vi "Main v2.vi"(0 "PID On":bool) -> (5 "Total (V)":dbl[](array[slide]) scale=-8.0..8.0, 6 "Force (N)":T2(graph)={"M1 ref force"=19.690402476780186, "M2 ref force"=19.690402476780186, "M1 mes force"=5.466389475814116, "M2 mes force"=1.4423805363163493})   [LabVIEW 2021]
uses:
  <vilib>/addons/control/pid/NI_PID_pid.lvlib
  <vilib>/platform/TimedLoop/XDataNode/XDataNode.xnode
  <vilib>/Platform/TimedLoop/XDataNode/nitl_modes.ctl
  <vilib>/Platform/TimedLoop/XDataNode/XDNodeRunTimeDep.lvlib
  <vilib>/Platform/TimedLoop/XDataNode/wakeup.ctl
  <vilib>/Platform/TimedLoop/XDataNode/timing_clust.ctl
  <vilib>/Analysis/NI_AALBase.lvlib
  <vilib>/DAQmx/configure/timing.llb/DAQmx Timing (Sample Clock).vi
  <vilib>/DAQmx/create/channels.llb/DAQmx Create Channel (DO-Digital Output).vi
  <vilib>/DAQmx/create/channels.llb/DAQmx Create Channel (AO-Voltage-Basic).vi
  <vilib>/DAQmx/create/channels.llb/DAQmx Create Channel (AI-Voltage-Basic).vi
  <vilib>/Analysis/baseanly.llb/Real Dot Product.vi
  <vilib>/DAQmx/write.llb/DAQmx Write (Digital 1D Bool 1Chan 1Samp).vi
  <vilib>/DAQmx/write.llb/DAQmx Write (Analog 1D DBL NChan 1Samp).vi
  <vilib>/addons/control/pid/pid.llb/PID (DBL).vi
panel:
  out "Period":i64
  out "Finished Late? [i-1]":bool
  in  "operation (0:open)":T1(ring)
  in  "Tab Control 2":enum32{"Start", "Trajectory", "RBF"}(tab)
  in  "Encoder":bool
  in  "Loadcell":bool
  in  "Set Tension":dbl=7.0
  in  "Motor Enable":bool[](array[boolean])=[FALSE, FALSE]
  in  "x":cluster{"Number":i32, "x_0":dbl, "x_f":dbl}={"Number"=20, "x_0"=0.0, "x_f"=500.0}
  in  "RBF":cluster{"STD":dbl, "Number":i32}={"STD"=150.0, "Number"=3}
  out "Weights":dbl[](array[numeric])=[3.49, 8.71, 7.36]
  out "Output":dbl(slide)=5.690310910676771 scale=0.0..10.0
  in  "Traj Start":i32(knob) scale=0.0..2.0
  in  "Tab Control":enum32{"Page 1", "Page 2"}(tab)
  out "XY Graph":cluster{dbl[], dbl[]}[](graph)=[{[0.0, 26.31578947368421, 52.63157894736842, 78.94736842105263, 105.26315789473684, 131.57894736842104, 157.89473684210526, 184.21052631578945, 210.52631578947367, 236.8421052631579, 263.1578947368421, 289.4736842105263, 315.7894736842105, 342.10526315789474, 368.4210526315789, 394.7368421052631, 421.05263157894734, 447.36842105263156, 473.6842105263158, 499.99999999999994], [3.49, 3.4367023266816097, 3.2816434014183695, 3.038602121132399, 2.728282054650678, 2.375405053956736, 2.0054833734466047, 1.6418498415053318, 1.303409208366113, 1.0033700058366293, 0.7489872481878055, 0.5421515616003525, 0.3805397094919775, 0.25900743528896036, 0.1709454164658713, 0.10940462192952286, 0.06789641734177898, 0.040859309931447936, 0.023843399552483855, 0.013492061286760112]}, {[0.0, 26.31578947368421, 52.63157894736842, 78.94736842105263, 105.26315789473684, 131.57894736842104, 157.89473684210526, 184.21052631578945, 210.52631578947367, 236.8421052631579, 263.1578947368421, 289.4736842105263, 315.7894736842105, 342.10526315789474, 368.4210526315789, 394.7368421052631, 421.05263157894734, 447.36842105263156, 473.6842105263158, 499.99999999999994], [2.1718577384502504, 2.86506550054527, 3.664972461281408, 4.546109122932967, 5.4681696051074065, 6.377890766498874, 7.213485399786169, 7.9112701950597755, 8.413568935864594, 8.676554069284796, 8.676554069284796, 8.413568935864594, 7.911270195059776, 7.213485399786169, 6.377890766498877, 5.468169605107408, 4.546109122932969, 3.6649724612814083, 2.86506550054527, 2.1718577384502518]}, {[0.0, 26.31578947368421, 52.63157894736842, 78.94736842105263, 105.26315789473684, 131.57894736842104, 157.89473684210526, 184.21052631578945, 210.52631578947367, 236.8421052631579, 263.1578947368421, 289.4736842105263, 315.7894736842105, 342.10526315789474, 368.4210526315789, 394.7368421052631, 421.05263157894734, 447.36842105263156, 473.6842105263158, 499.99999999999994], [0.028453172226519864, 0.050282928569135, 0.08616748455457215, 0.14318556780386613, 0.23072149495738908, 0.3605038009136996, 0.5462162532168332, 0.8025135420805027, 1.1433339522574764, 1.5795261165221341, 2.1159894678961577, 2.748736897872375, 3.462468433661673, 4.22932883340029, 5.009450199748302, 5.753626338747561, 6.408054903018468, 6.920600411014096, 7.247601468302764, 7.36]}, {[0.0, 26.31578947368421, 52.63157894736842, 78.94736842105263, 105.26315789473684, 131.57894736842104, 157.89473684210526, 184.21052631578945, 210.52631578947367, 236.8421052631579, 263.1578947368421, 289.4736842105263, 315.7894736842105, 342.10526315789474, 368.4210526315789, 394.7368421052631, 421.05263157894734, 447.36842105263156, 473.6842105263158, 499.99999999999994], [5.690310910676771, 6.352050755796014, 7.03278334725435, 7.727896811869232, 8.427173154715474, 9.11379962136931, 9.765185026449608, 10.35563357864561, 10.860312096488185, 11.259450191643559, 11.54153078536876, 11.704457395337322, 11.754278338213426, 11.701821668475418, 11.55828638271305, 11.331200565784492, 11.022060443293217, 10.626432182226953, 10.136510368400518, 9.545349799737012]}]
  out "Position (mm)":cluster{"Position":dbl, "ref_x (mm)":dbl}(graph)={"Position"=75.7275182286212, "ref_x (mm)"=0.0}
  in  "RBF":bool
  out "Speed (RPM)":dbl[](array[knob]) scale=-200.0..200.0
  in  "Set Point":dbl(slide)=19.690402476780186 scale=0.0..40.0
  in  "stop":bool
  in  "Tab Control 3":enum32{"Page 1", "Page 3", "Page 4", "Page 2"}(tab)=enum."Page 2"
  in  "PID gains":T3 {"derivative time (Td, min)" format="%.3f"; "integral time (Ti, min)" format="%.3f"; "proportional gain (Kc)" format="%.3f"}
  in  "Pos Control":bool
  out "output":dbl(knob)=-0.0 scale=-40.0..40.0
  in  "Gains":T4(array[cluster])=[{"proportional gain (Kc)"=0.17, "integral time (Ti, min)"=0.0, "derivative time (Td, min)"=0.0}, {"proportional gain (Kc)"=0.17, "integral time (Ti, min)"=0.0, "derivative time (Td, min)"=0.0}] {"derivative time (Td, min)" format="%.3f"; "integral time (Ti, min)" format="%.3f"; "proportional gain (Kc)" format="%.3f"}
  out "PID (V)":dbl[](array[slide])=[2.4180822101642323, 1.0] scale=-8.0..8.0
  # "FORCE"
  # "TRAJECTORY"
  # "INITIALIZE"
  # "TUNE"
  # "MONITOR"
  # "DEVEL"
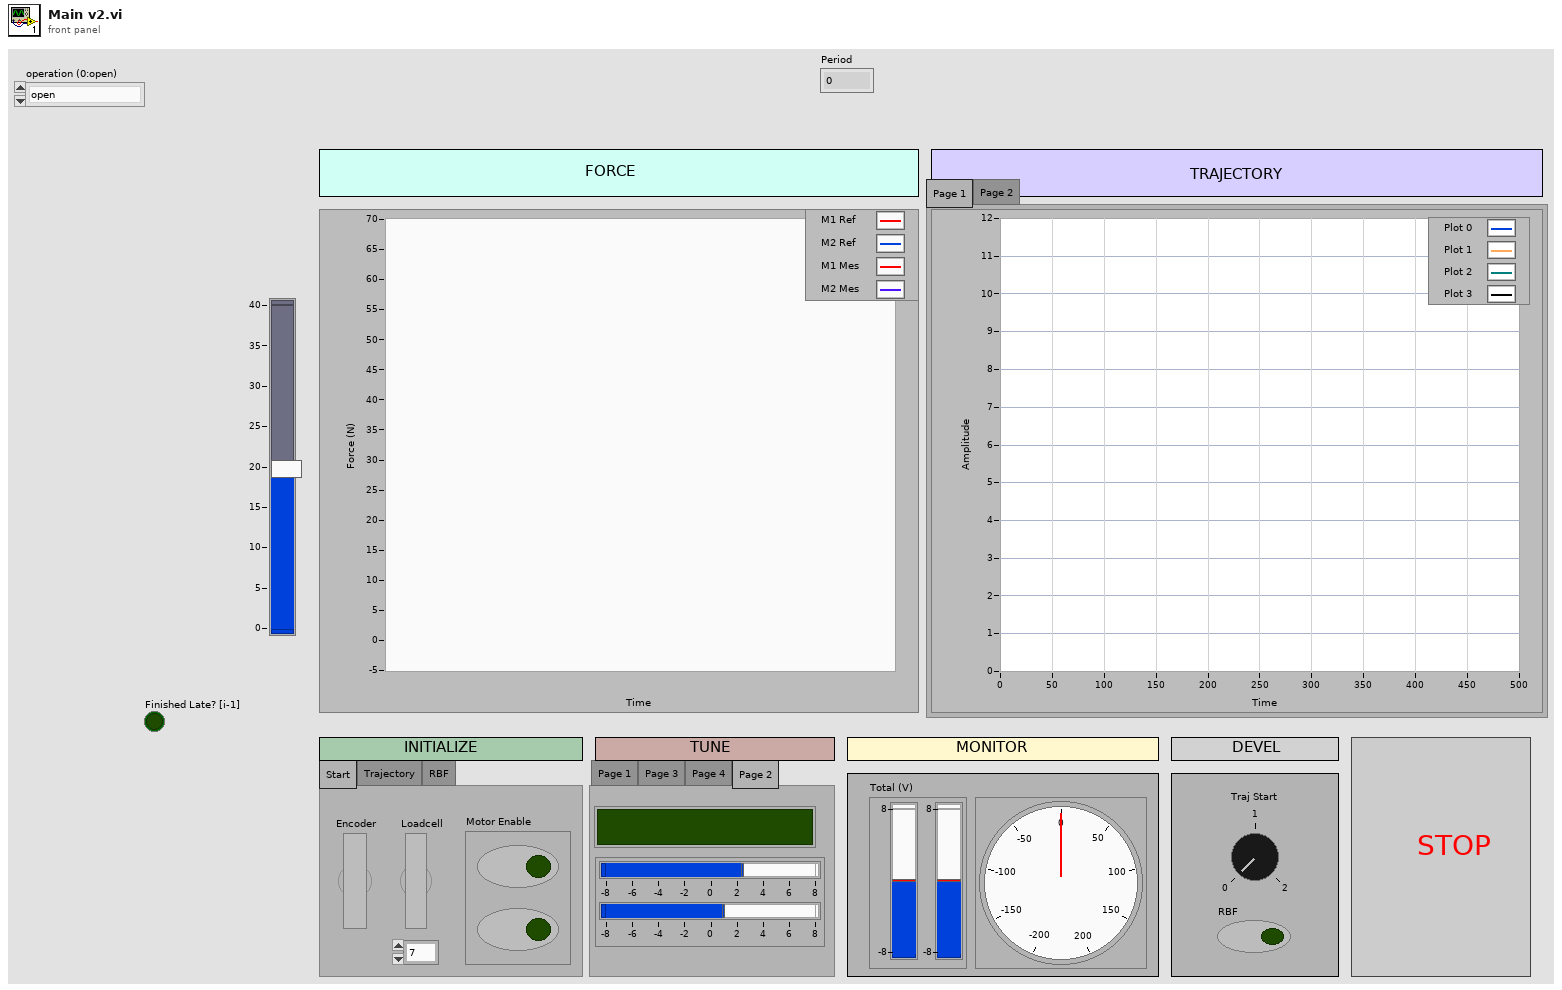
[diagram p1: front panel]
types:
  T1 = enum16{"open", "open or create", "create or replace", "create", "open (read-only)"}
  T2 = cluster{"M1 ref force":dbl, "M2 ref force":dbl, "M1 mes force":dbl, "M2 mes force":dbl}
  T3 = cluster{"proportional gain (Kc)":dbl, "integral time (Ti, min)":dbl, "derivative time (Td, min)":dbl}
  T4 = cluster{"proportional gain (Kc)":dbl, "integral time (Ti, min)":dbl, "derivative time (Td, min)":dbl}[]
  T5 = typedef "XDNodeRunTimeDep.lvlib/timing_clust.ctl" = cluster{"Expected End [f-1]":u64, "Actual End [f-1]":u64, "Finished Late? [f-1]":bool, "Expected End [i-1]":u64, "Actual End [i-1]":u64, "Finished Late? [i-1]":bool, "Expected Start [i]":u64, "Actual Start [i]":u64, "Expected Start [f]":u64, "Actual Start [f]":u64, "Source Name":string, "Structure Name":string, "Period":i64, "Deadline":i64, "Offset":i64, "Start":i64, "Priority":i32, "Timeout":i32, "Mode":T6, "Wakeup Reason":T7, "Error":errorcluster, "Source Type":string, "Secondary Source Type":string, "Global End Time":u64, "Global Start Time":u64, "Frame Duration":u64, "Iteration Duration":u64, "Assigned CPU":i32, "I/O Scan Engine Mode":u32}
  T6 = typedef "XDNodeRunTimeDep.lvlib/nitl_modes.ctl" = enum32{"No Change", "Process missed periods, maintain original phase", "Discard missed periods, maintain original phase", "Process missed periods, ignore original phase", "Discard missed periods, ignore original phase"}
  T7 = typedef "XDNodeRunTimeDep.lvlib/wakeup.ctl" = enum32{"Normal", "Aborted", "Asynchronous wakeup", "Timing source error", "Timed loop error", "Timeout"}
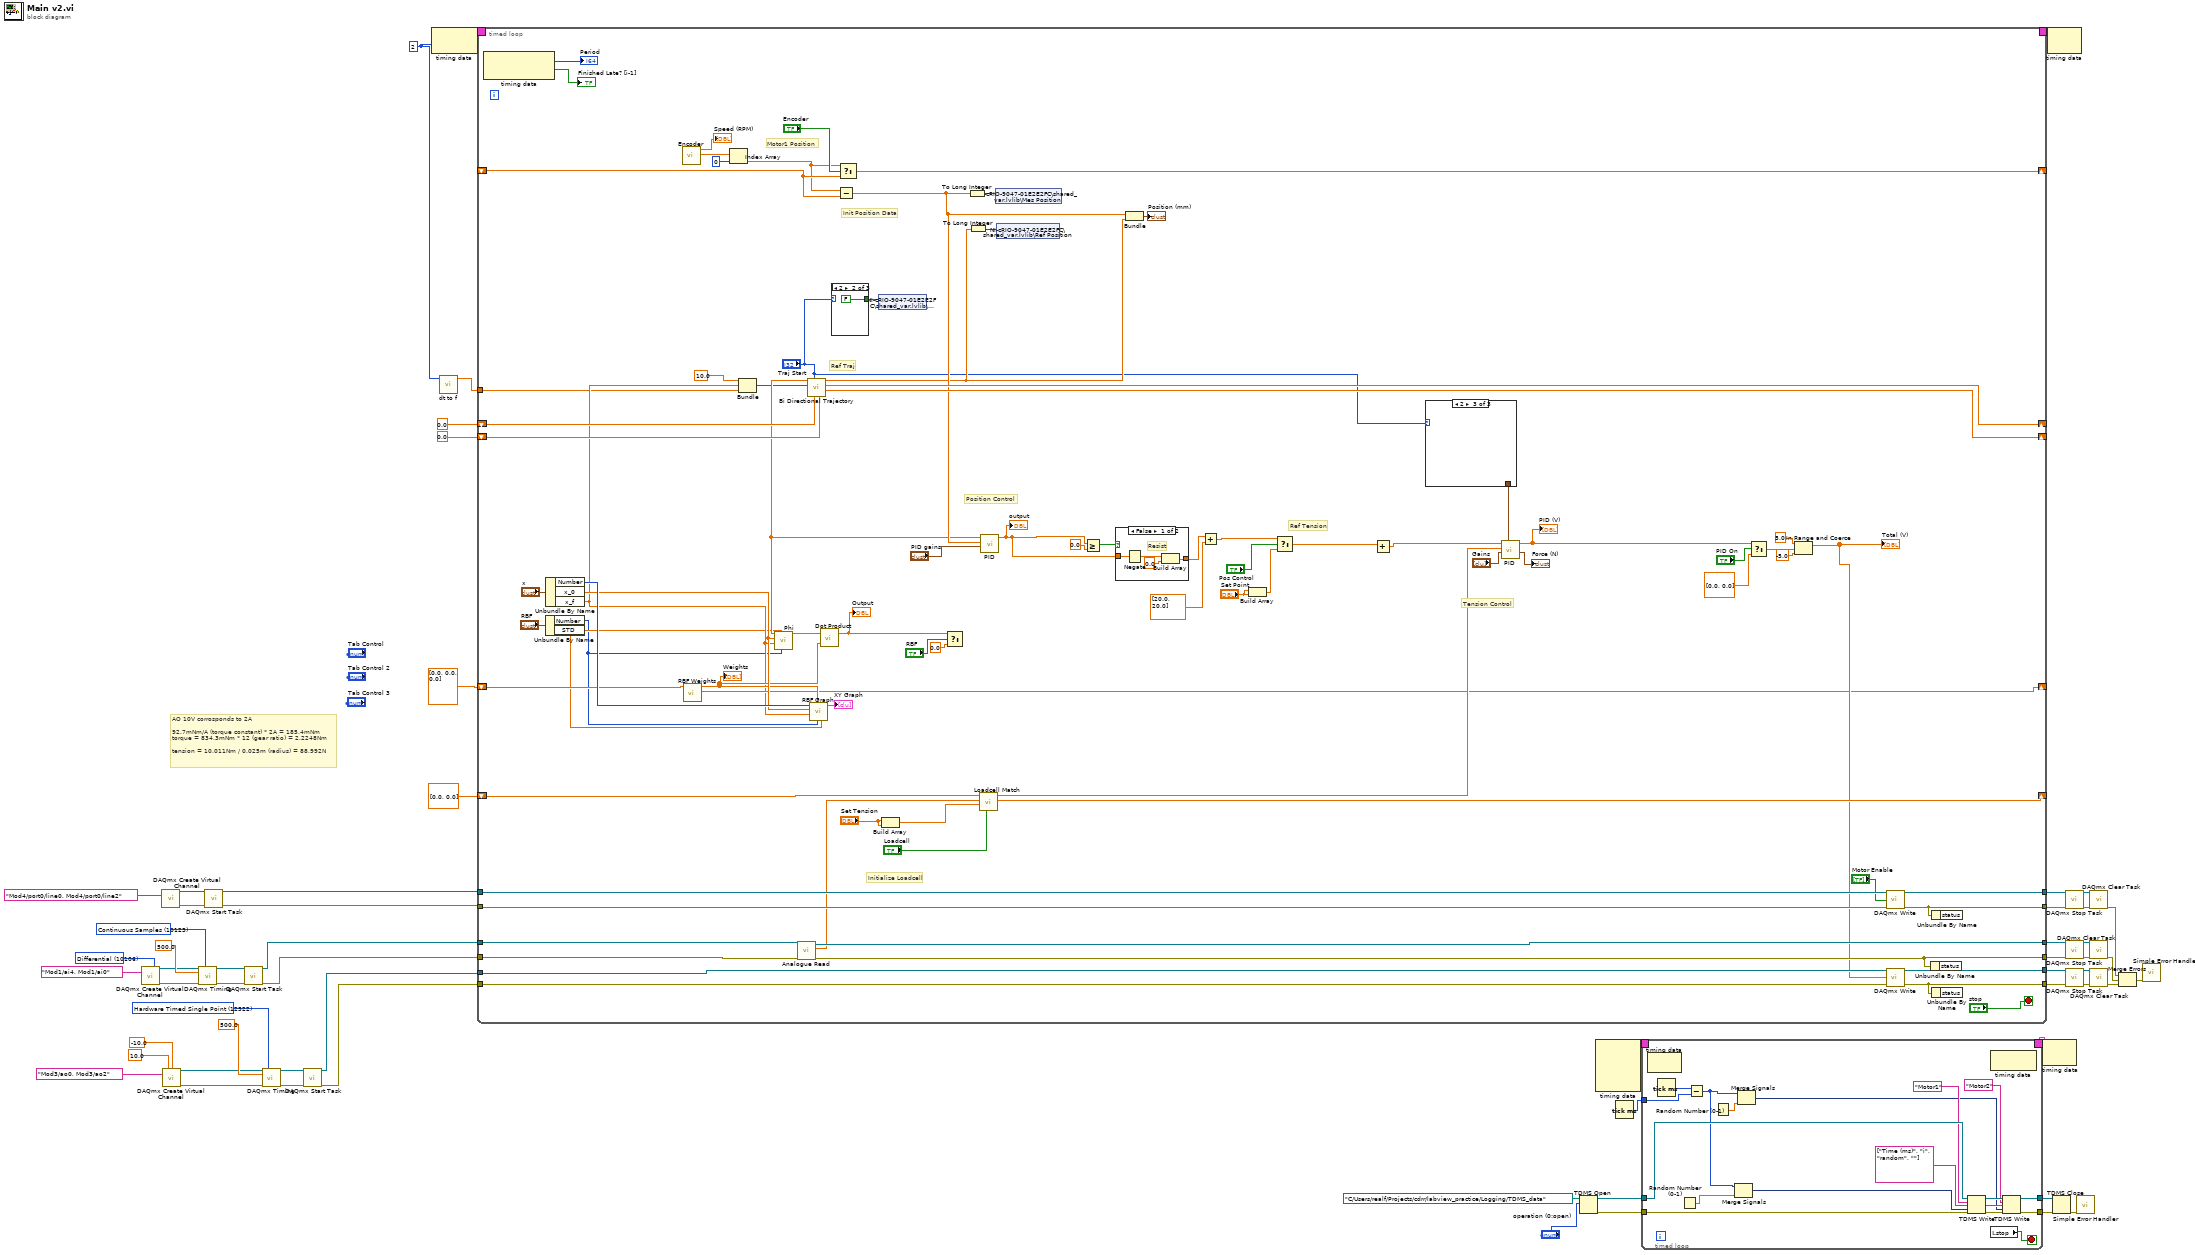
[diagram p0: block diagram]
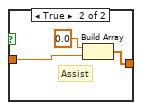
[diagram p2: hidden frame]
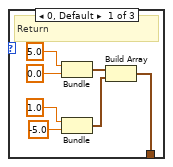
[diagram p3: hidden frame]
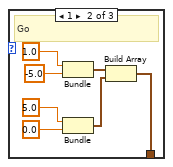
[diagram p4: hidden frame]
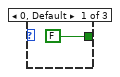
[diagram p5: hidden frame]
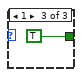
[diagram p6: hidden frame]
diagram:
  w15 = 12522 items=["Finite Samples"=10178, "Continuous Samples"=10123, "Hardware Timed Single Point"=12522] ("sample mode")
  w18 = 10123 items=["Finite Samples"=10178, "Continuous Samples"=10123, "Hardware Timed Single Point"=12522] ("sample mode")
  w25 = i64 2 ("Period")
  w32 = 10106 items=["Default"=-1, "RSE"=10083, "NRSE"=10078, "Differential"=10106, "Pseudodifferential"=12529] ("input terminal configuration")
  # "AO 10V corrosponds to 2A\n\n92.7mNm/A (torque constant) * 2A = 185.4mNm\ntorque = 834.3mNm * 12 (gear ratio) = 2.2248Nm\n\ntension = 10.011Nm / 0.025m (radius) = 88.992N"
  n1 = call-poly <vilib>:"DAQmx Create Virtual Channel.vi"("input terminal configuration"=w32, "physical channels"=tag "Mod1/ai4, Mod1/ai0") -> ("task out"=w22:refnum<k21>, "error out"=w21:errorcluster)  [unwired: 12 in]
  n2 = call-poly <vilib>:"DAQmx Create Virtual Channel.vi"("lines"=tag "Mod4/port0/line0, Mod4/port0/line2") -> ("task out"=w17:refnum<k21>, "error out"=w54:errorcluster)  [unwired: 13 in]
  n3 = call-poly <vilib>:"DAQmx Create Virtual Channel.vi"("maximum value"=10.0 ("AO max"), "minimum value"=-10.0 ("AO min"), "physical channels"=tag "Mod3/ao0, Mod3/ao2" ("Physical Channel(s)")) -> ("task out"=w14:refnum<k21>, "error out"=w12:errorcluster)  [unwired: 11 in]
  n4 = call-poly <vilib>:"DAQmx Timing.vi"("task/channels in"=w22, "sample mode"=w18, "rate"=500.0, "error in"=w21) -> ("task out"=w19:refnum<k21>, "error out"=w20:errorcluster)  [unwired: 10 in]
  n5 = call <vilib>:"DAQmx Start Task.vi"("task/channels in"=w17, "error in"=w54) -> ("task out"=w52:refnum<k21>, "error out"=w51:errorcluster)  [unwired: 12 in]
  n6 = call <vilib>:"DAQmx Start Task.vi"("task/channels in"=w19, "error in"=w20) -> ("task out"=w45:refnum<k21>, "error out"=w44:errorcluster)  [unwired: 12 in]
  n7 = call-poly <vilib>:"DAQmx Timing.vi"("task/channels in"=w14, "sample mode"=w15, "rate"=500.0, "error in"=w12) -> ("task out"=w13:refnum<k21>, "error out"=w11:errorcluster)  [unwired: 10 in]
  n8 = call <vilib>:"DAQmx Start Task.vi"("task/channels in"=w13, "error in"=w11) -> ("task out"=w56:refnum<k21>, "error out"=w55:errorcluster)  [unwired: 12 in]
  n9 = node-c288(w25) -> (w28:T5)
  n10 = call "dt to f.vi"("Period"=w25) -> ("Frequency"=w24:dbl)  [unwired: 10 in]
  n11 = timed-loop {
    tunnel: [w141] -> w60
    tunnel: [w140] -> w59
    tunnel: [w127] -> w58
    tunnel: [w132] -> w57
    tunnel: w45 -> [w138]
    tunnel: w44 -> [w137]
    tunnel: w56 -> [w126]
    tunnel: w55 -> [w139]
    tunnel: w52 -> [w136]
    tunnel: w51 -> [w135]
    tunnel: [w134] -> w48
    tunnel: [w133] -> w47
    shift-right: [w130] -> _
    shift-left: 0.0 ("total time") -> [w131]
    shift-right: [w129] -> _
    shift-left: _ -> [w128]
    shift-right: [w124] -> _
    shift-left: dbl[] [0.0, 0.0] ("measured force") -> [w125]
    shift-right: [w122] -> _
    shift-left: 0.0 ("total time") -> [w123]
    timing: w28 -> [_]
    timing-out: [_] -> w27
    shift-right: [w78] -> _
    shift-left: dbl[] [0.0, 0.0, 0.0] ("Array of Double") -> [w79]
    tunnel: w24 -> [w70]
    stop <- "stop" stop-if-true
    # "Initialize Loadcell"
    # "Tension Control"
    # "Ref Tension"
    # "Position Control"
    # "Ref Traj"
    # "Init Position Data"
    # "Motor1 Position"
    n12 = node-c288() -> (→"Period":i64, →"Finished Late? [i-1]":bool)  [unwired: 1 in]
    n13 = Unbundle By Name("RBF") -> ("Number"=w66:i32, "STD"=w67:dbl)
    n14 = Unbundle By Name("x") -> ("Number"=w88:i32, "x_0"=w85:dbl, "x_f"=w71:dbl)
    n15 = call "Encoder.vi"() -> ("Mes Pos (mm)"=w92:dbl[], "RPM"=→"Speed (RPM)":dbl[])  [unwired: 10 in]
    n16 = call "RBF Weights.vi"("Array of Double in"=w79) -> ("Array of Double out"=w78:dbl[], "Array of Double 3"=w80:dbl[])  [unwired: 9 in]
    "Weights" <- w80
    n17 = Index Array(array=w92, index=0) -> (element=w104:dbl)
    n18 = Bundle("y"=10.0, "x_f"=w71, "Frequency"=w70) -> (w69:cluster{"y":dbl, "x_f":dbl, "Frequency":dbl})  [unwired: 1 in]
    n19 = call "Analogue Read.vi"("error in"=w137, "task/channels in"=w138) -> ("error out"=w132:errorcluster, "measured force"=w100:dbl[], "task out"=w127:refnum<k21>)  [unwired: 6 in, 1 out]
    n20 = call "Bi Directional Trajectory.vi"("Return Time"=w123, "Go Time"=w131, "Traj Start"="Traj Start", "Trajectory Settings"=w69) -> ("Return Next Time"=w122:dbl, "Go Next Time"=w130:dbl, "Output (mm)"=w84:dbl)  [unwired: 5 in]
    n21 = call "Phi.vi"("Number"=w66, "STD"=w67, "x_f"=w71, "x_0"=w85, "Output (mm)"=w84) -> ("Array"=w83:dbl[])  [unwired: 6 in]
    n22 = call "RBF Graph.vi"("STD"=w67, "Number"=w66, "Array of Double 3"=w80, "x_f"=w71, "x_0"=w85, "Number 2"=w88) -> ("Array"=→"XY Graph":cluster{dbl[], dbl[]}[])  [unwired: 5 in]
    n23 = call-poly <vilib>:"Dot Product.vi"("Y Vector"=w80, "X Vector"=w83) -> ("X * Y"=w77:dbl)  [unwired: 1 out]
    "Output" <- w77
    n24 = case shown="2" "Traj Start" {
      tunnel: [FALSE FALSE TRUE] -> w81
      frame 0, Default {
      }
      frame 2 {
      }
      frame 1 {
      }
    }
    n25 = Subtract(x=w104, y=w128) -> (x-y=w106:dbl)
    n26 = Select(t=w104, s="Encoder", f=w128) -> (s? t:f=w129:dbl)
    n27 = shared-variable "NI-cRIO-9047-01E2E2FC\\shared_var.lvlib\\Trigger"(w81) -> ()  [unwired: 1 in, 1 out]
    n28 = Build Array("Set Tension", "Set Tension") -> (w98:dbl[])
    n29 = Select(t=w77, s="RBF", f=0.0) -> ()  [unwired: 1 out]
    n30 = To Long Integer(number=w106) -> (32bit integer=w94:i32)
    n31 = To Long Integer(number=w84) -> (32bit integer=w95:i32)
    n32 = call "Loadcell Match.vi"("Initialize"="Loadcell", "Set Tension"=w98, "Mes Tension"=w100, "Next Tension Error"=w125) -> ("Tension Error"=w124:dbl[], "Filtered Tension"=w108:dbl[])  [unwired: 6 in]
    n33 = call-poly <vilib>:"PID.vi"("PID gains"="PID gains", "process variable"=w106, "setpoint"=w84) -> ("output"=w63:dbl)  [unwired: 7 in, 1 out]
    "output" <- w63
    n34 = shared-variable "NI-cRIO-9047-01E2E2FC\\shared_var.lvlib\\Mes Position"(w94) -> ()  [unwired: 1 in, 1 out]
    n35 = shared-variable "NI-cRIO-9047-01E2E2FC\\shared_var.lvlib\\Ref Position"(w95) -> ()  [unwired: 1 in, 1 out]
    n36 = Greater Or Equal?(x=w63, y=0.0) -> (x >= y?=w76:bool)
    n37 = case shown="False" w76 {
      tunnel: w63 -> [w147 w150]
      tunnel: [w148 w151] -> w73
      frame False {
        # "Resist"
        n38 = Negate(x=w147) -> (-x=w145:dbl)
        n39 = Build Array(w145, 0.0 ("element")) -> (w148:dbl[])
      }
      frame True {
        # "Assist"
        n40 = Build Array(0.0 ("element"), w150) -> (w151:dbl[])
      }
    }
    n41 = Bundle(w106, "Output (mm)"=w84) -> (→"Position (mm)":cluster{dbl, "Output (mm)":dbl})  [unwired: 1 in]
    n42 = Add(x=w73, y=dbl[] [20.0, 20.0] ("x")) -> (x+y=w72:dbl[])
    n43 = Build Array("Set Point", "Set Point") -> (w114:dbl[])
    n44 = Select(t=w72, s="Pos Control", f=w114) -> (s? t:f=w62:dbl[])
    n45 = Add(x=w62) -> (x+y=w61:dbl[])  [unwired: 1 in]
    n46 = case shown="2" "Traj Start" {
      tunnel: [w152 w159 _] -> w109
      frame 0, Default {
        # "Return"
        n47 = Bundle(5.0, 0.0) -> (w158:cluster{dbl, dbl})  [unwired: 1 in]
        n48 = Bundle(1.0, -5.0) -> (w157:cluster{dbl, dbl})  [unwired: 1 in]
        n49 = Build Array(w158, w157) -> (w152:cluster{dbl, dbl}[])
      }
      frame 1 {
        # "Go"
        n50 = Bundle(1.0, -5.0) -> (w160:cluster{dbl, dbl})  [unwired: 1 in]
        n51 = Bundle(5.0, 0.0) -> (w161:cluster{dbl, dbl})  [unwired: 1 in]
        n52 = Build Array(w160, w161) -> (w159:cluster{dbl, dbl}[])
      }
      frame 2 {
      }
    }
    n53 = call <vilib>:"PID.vi"("output range"=w109, "PID gains"="Gains", "mes force"=w108, "ref force"=w61) -> ("output cluster"=→"Force (N)":T2, "PID output"=w118:dbl[])  [unwired: 6 in]
    "PID (V)" <- w118
    n54 = Select(t=w118, s="PID On", f=dbl[] [0.0, 0.0]) -> (s? t:f=w116:dbl[])
    n55 = In Range and Coerce(upper limit=5.0, x=w116, lower limit=-5.0) -> (coerced(x)=w96:dbl[])  [unwired: 1 out]
    "Total (V)" <- w96
    n56 = call-poly <vilib>:"DAQmx Write.vi"("task/channels in"=w136, "data"="Motor Enable", "error in"=w135) -> ("task out"=w134:refnum<k21>, "error out"=w133:errorcluster)  [unwired: 10 in, 1 out]
    n57 = call-poly <vilib>:"DAQmx Write.vi"("task/channels in"=w126, "data"=w96, "error in"=w139) -> ("task out"=w141:refnum<k21>, "error out"=w140:errorcluster)  [unwired: 10 in, 1 out]
    n58 = Unbundle By Name(w132) -> ()  [unwired: 1 out]
    n59 = Unbundle By Name(w133) -> ()  [unwired: 1 out]
    n60 = Unbundle By Name(w140) -> ()  [unwired: 1 out]
  }
  n61 = TDMS Open(10:"operation (0:open)", 11:path "C:/Users/realf/Projects/cdrr/labview_practice/Logging/TDMS_data" ("file path")) -> (0:w6:errorcluster, 3:w10:refnum<k34>)  [unwired: 5 in]
  n62 = node-c288() -> (w2:T5)  [unwired: 4 in]
  n63 = Tick Count (ms)() -> (millisecond timer value=w3:u32)
  n64 = timed-loop {
    tunnel: w10 -> [w187]
    tunnel: [w181] -> w9
    tunnel: [w183] -> w7
    tunnel: w6 -> [w186]
    tunnel: w3 -> [w172]
    timing: w2 -> [_]
    timing-out: [_] -> w1
    stop <- w170 stop-if-true
    n65 = node-c288() -> ()  [unwired: 1 in, 1 out]
    n66 = Tick Count (ms)() -> (millisecond timer value=w174:u32)
    n67 = Random Number (0-1)() -> (number: 0 to 1=w173:dbl)
    n68 = Subtract(x=w174, y=w172) -> (x-y=w171:u32)
    n69 = Random Number (0-1)() -> (number: 0 to 1=w176:dbl)
    n70 = Merge Signals(w171, w173) -> (w177:dynamicdata)  [unwired: 1 in]
    n71 = Merge Signals(w171, w176) -> (w175:dynamicdata)  [unwired: 1 in]
    n72 = TDMS Write(0:w187, 5:"Motor1" ("group name in (Untitled)"), 7:string[] ["Time (ms)", "i", "random", ""] ("channel name(s) in (Untitled)"), 9:w177, 11:w186) -> (4:w182:refnum<k34>, 8:w178:string[], 15:w184:errorcluster)  [unwired: 1 in, 1 out]
    n73 = node-c288() -> ()  [unwired: 1 in, 1 out]
    n74 = local read "stop"() -> (w170:bool)
    n75 = TDMS Write(0:w182, 5:"Motor2" ("group name in (Untitled)"), 7:w178, 9:w175, 11:w184) -> (4:w181:refnum<k34>, 15:w183:errorcluster)  [unwired: 1 in, 2 out]
  }
  n76 = node-c288(w1) -> ()  [unwired: 1 out]
  n77 = node-c288(w27) -> ()  [unwired: 1 out]
  n78 = TDMS Close(8:w7, 11:w9) -> (0:w8:errorcluster)  [unwired: 1 out]
  n79 = call <vilib>:"DAQmx Stop Task.vi"("task/channels in"=w48, "error in"=w47) -> ("task out"=w50:refnum<k21>, "error out"=w49:errorcluster)  [unwired: 12 in]
  n80 = call <vilib>:"DAQmx Stop Task.vi"("task/channels in"=w58, "error in"=w57) -> ("task out"=w38:refnum<k21>, "error out"=w37:errorcluster)  [unwired: 12 in]
  n81 = call <vilib>:"DAQmx Stop Task.vi"("task/channels in"=w60, "error in"=w59) -> ("task out"=w40:refnum<k21>, "error out"=w39:errorcluster)  [unwired: 12 in]
  n82 = call <vilib>:"Simple Error Handler.vi"("error in (no error)"=w8) -> ()  [unwired: 4 in, 5 out]
  n83 = call <vilib>:"DAQmx Clear Task.vi"("task in"=w50, "error in"=w49) -> ("error out"=w33:errorcluster)  [unwired: 13 in]
  n84 = call <vilib>:"DAQmx Clear Task.vi"("task in"=w38, "error in"=w37) -> ("error out"=w34:errorcluster)  [unwired: 13 in]
  n85 = call <vilib>:"DAQmx Clear Task.vi"("task in"=w40, "error in"=w39) -> ("error out"=w35:errorcluster)  [unwired: 13 in]
  n86 = Merge Errors(w33, w34, w35) -> (w36:errorcluster)
  n87 = call <vilib>:"Simple Error Handler.vi"("error in (no error)"=w36) -> ()  [unwired: 4 in, 5 out]
